vi "Add User Channel_Channel.vi"(8 "error in":errorcluster, 10 "User Channel Settings":T1, 11 "User Ref":refnum<k24>) -> (0 "error out":errorcluster, 3 "User Ref out":refnum<k24>)   [LabVIEW 2019, in "Simple SysDef API.lvlib"]
uses:
  <userlib>/SimpleSysDef/Simple SysDef API.lvlib
  NationalInstruments.VeriStand.SystemDefinitionAPI
  <userlib>/SimpleSysDef/_SubVIs/Add User Channel_Settings.ctl
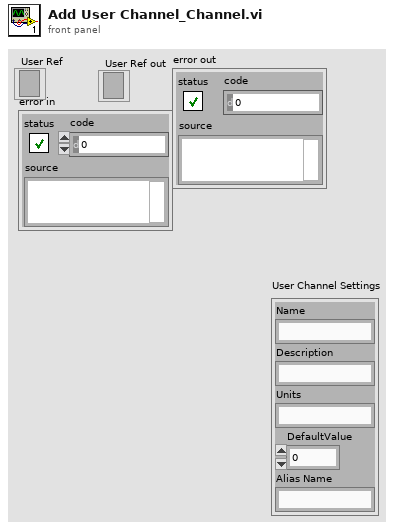
[diagram p1: front panel]
types:
  T1 = typedef "Simple SysDef API.lvlib/Add User Channel_Settings.ctl" = cluster{"Name":string, "Description":string, "Units":string, "DefaultValue":dbl, "Alias Name":string}
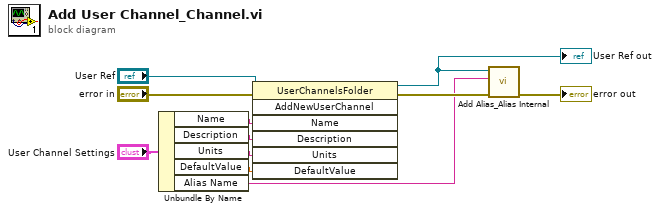
[diagram p0: block diagram]
diagram:
  n1 = Unbundle By Name("User Channel Settings") -> ("Name"=w8:string, "Description"=w7:string, "Units"=w6:string, "DefaultValue"=w5:dbl, "Alias Name"=w2:string)
  n2 = invoke class="UserChannelsFolder" method="AddNewUserChannel"(reference="User Ref", error in="error in", "Name"=w8, "Description"=w7, "Units"=w6, "DefaultValue"=w5) -> (reference out=w1:refnum<k24>, error out=w4:errorcluster)  [unwired: 1 in, 5 out]
  "User Ref out" <- w1
  n3 = call <userlib>:"Add Alias_Alias Internal.vi"("error in (no error)"=w4, "Name"=w2, "Base Node"=w1) -> ("error out"=→"error out":errorcluster)  [unwired: 7 in, 1 out]
